vi "Serialize as VTT.vi"(8 "error in (no error)":errorcluster, 11 "Element in":refnum<class "Element.lvclass">) -> (0 "error out":errorcluster, 2 "VTT Fragment":string, 3 "Element out":refnum<class "Element.lvclass">)   [LabVIEW 2023, in "VILab.lvlib" / "Element.lvclass"]
uses:
  Element.lvclass
  Element.lvclass/Element.ctl
  Attribute/Attribute.lvclass
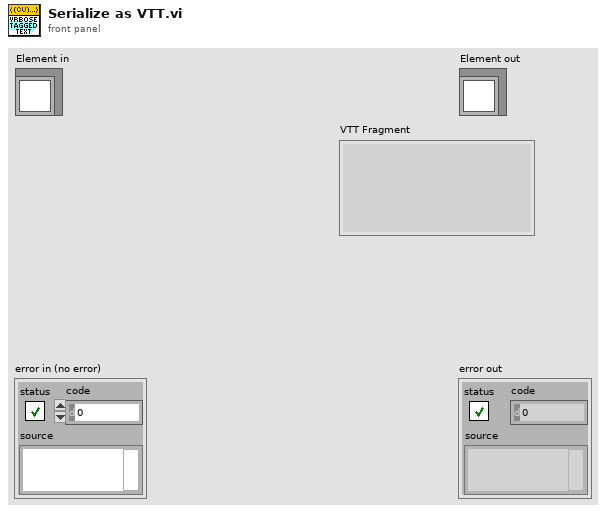
[diagram p1: front panel]
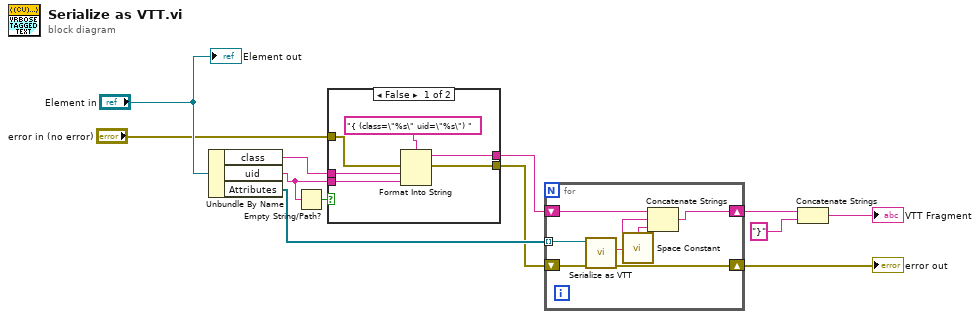
[diagram p0: block diagram]
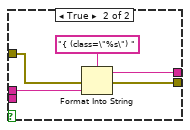
[diagram p2: hidden frame]
diagram:
  n1 = Unbundle By Name("Element in") -> ("class"=w10:string, "uid"=w2:string, "Attributes"=w11:refnum<class "Attribute.lvclass">[])
  n2 = Empty String/Path?(string/path=w2) -> (empty?=w1:bool)
  n3 = case shown="False" w1 {
    tunnel: w10 -> [w17 w22]
    tunnel: w2 -> [w16 _]
    tunnel: "error in (no error)" -> [w15 w21]
    tunnel: [w14 w20] -> w8
    tunnel: [w13 w19] -> w7
    frame False {
      n4 = Format Into String(format string="{ (class=\"%s\" uid=\"%s\") ", error in=w15, w17, w16) -> (resulting string=w13:string, error out=w14:errorcluster)  [unwired: 1 in]
    }
    frame True {
      n5 = Format Into String(format string="{ (class=\"%s\") ", error in=w21, w22) -> (resulting string=w19:string, error out=w20:errorcluster)  [unwired: 1 in]
    }
  }
  n6 = for {
    tunnel: w11 -> [w30] mode=indexing
    shift-right: [w26] -> w6
    shift-left: w8 -> [w29]
    shift-right: [w27] -> w5
    shift-left: w7 -> [w28]
    n7 = call-dynamic "Serialize as VTT.vi"("error in (no error)"=w29, "Attribute in"=w30) -> ("error out"=w26:errorcluster, "VTT Fragment"=w25:string)  [unwired: 7 in, 1 out]
    n8 = call <vilib>:"Space Constant.vi"() -> ("String"=w24:string)
    n9 = Concatenate Strings(w28, w25, w24) -> (w27:string)
  }
  "error out" <- w6
  n10 = Concatenate Strings(w5, "}") -> (→"VTT Fragment":string)
  "Element out" <- "Element in"
